vi "Read Debug Mode.vi"(8 "error in (no error)":errorcluster, 11 "Instrument in":refnum<class "Instrument.lvclass">) -> (0 "error out":errorcluster, 2 "Debug Mode?":bool, 3 "Instrument out":refnum<class "Instrument.lvclass">)   [LabVIEW 2019, in "Instrument.lvlib" / "Instrument.lvclass"]
uses:
  Instrument.lvclass
  C:/Program Files (x86)/National Instruments/LabVIEW 2019/vi.lib/JKI/JKI SMO/SMO/SMO.lvclass
  <userlib>/LevyLab/Debug/Attribute.Debug/DebugBehavior.ctl
  <userlib>/LevyLab/Debug/Debug.lvlib
  <userlib>/LevyLab/Debug/Attribute.Debug/Attribute.Debug.lvclass
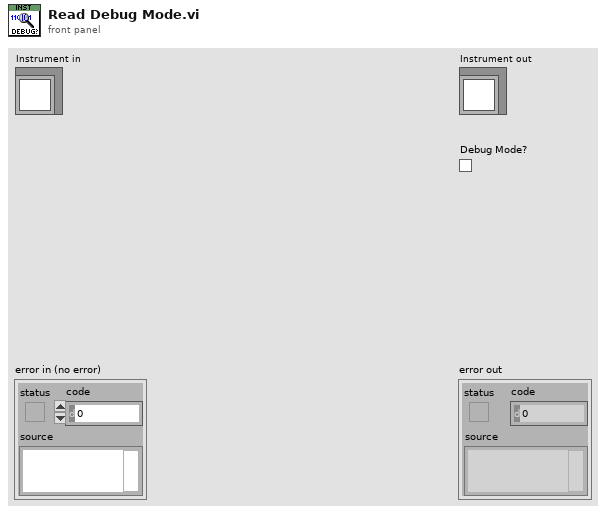
[diagram p1: front panel]
types:
  T1 = typedef "Debug.lvlib/Attribute.Debug.lvclass/DebugBehavior.ctl" = enum16{"Normal", "Debug"}
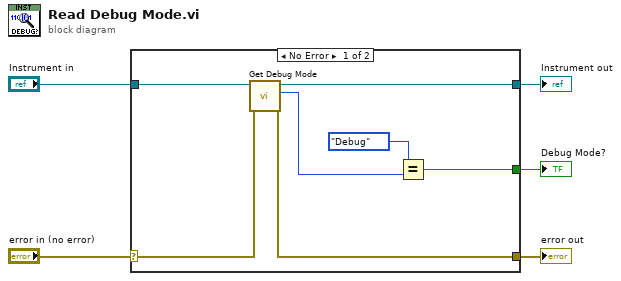
[diagram p0: block diagram]
diagram:
  n1 = case shown="No Error" "error in (no error)" {
    selector: "error in (no error)" -> [w7 w13]
    tunnel: [w6 w13] -> w4
    tunnel: [w12 w14] -> w2
    tunnel: "Instrument in" -> [w11 w14]
    tunnel: [w8 _] -> w1
    frame No Error {
      n2 = call <userlib>:"Get Debug Mode.vi"("error in (no error)"=w7, "SMO"=w11) -> ("error out"=w6:errorcluster, "Behavior"=w9:T1, "SMO out"=w12:refnum<class "Instrument.lvclass">)  [unwired: 7 in]
      n3 = Equal?(x=DebugBehavior."Debug" ("Behavior"), y=w9) -> (x = y?=w8:bool)
    }
    frame Error {
    }
  }
  "error out" <- w4
  "Instrument out" <- w2
  "Debug Mode?" <- w1
